vi "Test dropdown cell.vi"(11 "Test Case In":refnum<class "Test Cases.lvclass">) -> (0 "error out":errorcluster, 3 "Test Case Out":refnum<class "Test Cases.lvclass">)   [LabVIEW 2024, in "Test Cases.lvclass"]
uses:
  Test Cases.lvclass
  Test Cases.lvclass/Test Cases.ctl
  source/Grid/SourceGrid.lvclass
  <vilib>/Astemes/LUnit/Test Case.lvclass
  source/Cells/Cell/Cell.lvclass
  source/Views/Cell View/Cell View.lvclass
  source/System.Drawing.Color.ctl
  source/SourceGrid.lvlib
  source/Editors/Combo Box/Combo Box.lvclass
  C:/Program Files/National Instruments/LabVIEW 2025/vi.lib/Astemes/LUnit/Test Case.lvclass
  C:/Program Files/National Instruments/LabVIEW 2025/vi.lib/Astemes/LUnit/LUnit Runnable.lvclass
  D:/git/Sourcegrid-LabVIEW/tests/Tests/Test Cases.lvclass
  D:/git/Sourcegrid-LabVIEW/source/Editors/Editor Base/Editor Control Base.lvclass
  D:/git/Sourcegrid-LabVIEW/source/Editors/Combo Box/Combo Box.lvclass
  D:/git/Sourcegrid-LabVIEW/dll/SourceGrid.dll
  dll/SourceGrid.dll
panel:
  in  "stop":bool
  in  "Grid Container":refnum<k24>(container)
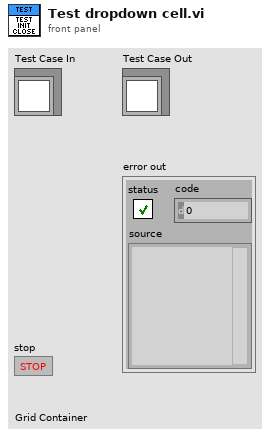
[diagram p1: front panel]
types:
  T1 = typedef "SourceGrid.lvlib/System.Drawing.Color.ctl" = enum16{"AliceBlue", "AntiqueWhite", "Aqua", "Aquamarine", "Azure", "Beige", "Bisque", "Black", "BlanchedAlmond", "Blue", "BlueViolet", "Brown", "BurlyWood", "CadetBlue", "Chartreuse", "Chocolate", "Coral", "CornflowerBlue", "Cornsilk", "Crimson", "Cyan", "DarkBlue", "DarkCyan", "DarkGoldenrod", "DarkGray", "DarkGreen", "DarkKhaki", "DarkMagenta", "DarkOliveGreen", "DarkOrange", "DarkOrchid", "DarkRed", "DarkSalmon", "DarkSeaGreen", "DarkSlateBlue", "DarkSlateGray", "DarkTurquoise", "DarkViolet", "DeepPink", "DeepSkyBlue", "DimGray", "DodgerBlue", "Firebrick", "FloralWhite", "ForestGreen", "Fuchsia", "Gainsboro", "GhostWhite", "Gold", "Goldenrod", "Gray", "Green", "GreenYellow", "Honeydew", "HotPink", "IndianRed", "Indigo", "Ivory", "Khaki", "Lavender", "LavenderBlush", "LawnGreen", "LemonChiffon", "LightBlue", "LightCoral", "LightCyan", "LightGoldenrodYellow", "LightGray", "LightGreen", "LightPink", "LightSalmon", "LightSeaGreen", "LightSkyBlue", "LightSlateGray", "LightSteelBlue", "LightYellow", "Lime", "LimeGreen", "Linen", "Magenta", "Maroon", "MediumAquamarine", "MediumBlue", "MediumOrchid", "MediumPurple", "MediumSeaGreen", "MediumSlateBlue", "MediumSpringGreen", "MediumTurquoise", "MediumVioletRed", "MidnightBlue", "MintCream", "MistyRose", "Moccasin", "NavajoWhite", "Navy", "OldLace", "Olive", "OliveDrab", "Orange", "OrangeRed", "Orchid", "PaleGoldenrod", "PaleGreen", "PaleTurquoise", "PaleVioletRed", "PapayaWhip", "PeachPuff", "Peru", "Pink", "Plum", "PowderBlue", "Purple", "Red", "RosyBrown", "RoyalBlue", "SaddleBrown", "Salmon", "SandyBrown", "SeaGreen", "SeaShell", "Sienna", "Silver", "SkyBlue", "SlateBlue", "SlateGray", "Snow", "SpringGreen", "SteelBlue", "Tan", "Teal", "Thistle", "Tomato", "Transparent", "Turquoise", "Violet", "Wheat", "White", "WhiteSmoke", "Yellow"}
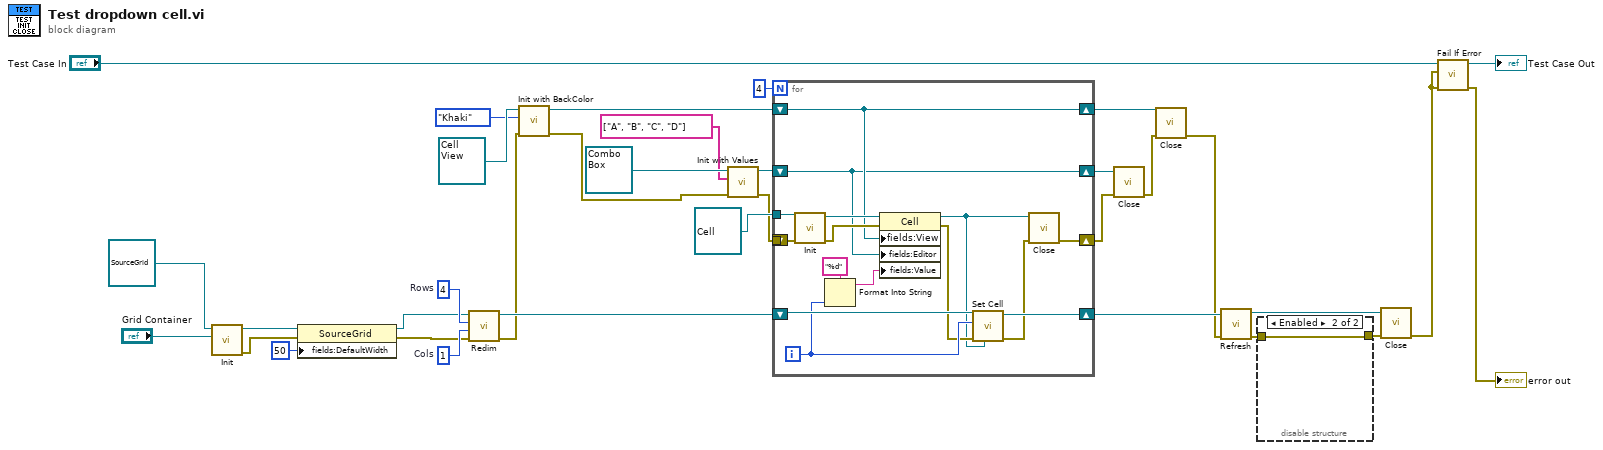
[diagram p0: block diagram]
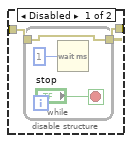
[diagram p2: hidden frame]
diagram:
  w30 = 1  # Cols
  w31 = 4  # Rows
  n1 = call-dynamic "Init.vi"("Sourcegrid Container"="Grid Container", "Grid in"=refnum<class "SourceGrid.lvclass"> refnum) -> ("error out"=w18:errorcluster, "Grid out"=w27:refnum<class "SourceGrid.lvclass">)  [unwired: 8 in]
  n2 = property class="SourceGrid"(reference=w27, error in=w18, "fields:DefaultWidth"=50 ("DefaultWidth")) -> (reference out=w26:refnum<class "SourceGrid.lvclass">, error out=w25:errorcluster)
  n3 = call "Redim.vi"("error in"=w25, "Columns"=w30, "Rows"=w31, "Sourcegrid in"=w26) -> ("error out"=w4:errorcluster, "Sourcegrid out"=w22:refnum<class "SourceGrid.lvclass">)  [unwired: 6 in]
  n4 = call-dynamic "Init with BackColor.vi"("error in"=w4, "Color"=System.Drawing.Color."Khaki", "Cell View in"=refnum<class "Cell View.lvclass"> refnum) -> ("error out"=w14:errorcluster, "Cell View out"=w6:refnum<class "Cell View.lvclass">)  [unwired: 7 in]
  n5 = call-dynamic "Init with Values.vi"("error in"=w14, "Values"=string[] ["A", "B", "C", "D"], "Combo Box in"=refnum<class "Combo Box.lvclass"> refnum ("SourceGrid.lvlib:Combo Box.lvclass")) -> ("error out"=w9:errorcluster, "Combo Box out"=w11:refnum<class "Combo Box.lvclass">)  [unwired: 7 in]
  n6 = for {
    N: 4 -> [_]
    shift-right: [w47] -> w3
    shift-left: _ -> [_]
    shift-right: [w49] -> w23
    shift-left: w22 -> [w48]
    tunnel: refnum<class "Cell.lvclass"> refnum ("Cell in") -> [w41]
    tunnel: w9 -> [w44]
    shift-right: [w37] -> w5
    shift-left: w6 -> [w37]
    shift-right: [w36] -> w1
    shift-left: w11 -> [w36]
    i -> [w45]
    n7 = call-dynamic "Init.vi"("error in"=w44, "Cell in"=w41) -> ("error out"=w39:errorcluster, "Cell out"=w40:refnum<class "Cell.lvclass">)  [unwired: 8 in]
    n8 = Format Into String(format string="%d", w45) -> (resulting string=w38:string)  [unwired: 2 in, 1 out]
    n9 = property class="Cell"(reference=w40, error in=w39, "fields:View"=w37, "fields:Editor"=w36, "fields:Value"=w38) -> (reference out=w35:refnum<class "Cell.lvclass">, error out=w42:errorcluster)
    n10 = call "Set Cell.vi"("Cell"=w35, "error in"=w42, "Row"=w45, "Sourcegrid in"=w48) -> ("error out"=w43:errorcluster, "Sourcegrid out"=w49:refnum<class "SourceGrid.lvclass">)  [unwired: 6 in]
    n11 = call-dynamic "Close.vi"("error in"=w43, "Cell in"=w35) -> ("error out"=w47:errorcluster)  [unwired: 8 in, 1 out]
  }
  n12 = call-dynamic "Close.vi"("error in"=w3, "Combo Box in"=w1) -> ("error out"=w2:errorcluster)  [unwired: 8 in, 1 out]
  n13 = call-dynamic "Close.vi"("error in"=w2, "Cell View in"=w5) -> ("error out"=w13:errorcluster)  [unwired: 8 in, 1 out]
  n14 = call "Refresh.vi"("error in"=w13, "SourceGrid in"=w23) -> ("error out"=w8:errorcluster, "SourceGrid out"=w20:refnum<class "SourceGrid.lvclass">)  [unwired: 8 in]
  n15 = disable-structure shown="Enabled" {
    disable-tunnel: w8 -> [w51 w55]
    disable-tunnel: [w50 w55] -> w7
    frame Disabled {
      n16 = while {
        tunnel: w51 -> [w52]
        tunnel: [w52] -> w50
        stop <- "stop" stop-if-true
        n17 = Wait (ms)(milliseconds to wait=u32 1) -> ()  [unwired: 1 out]
      }
    }
    frame Enabled {
    }
  }
  n18 = call-dynamic "Close.vi"("error in"=w7, "Sourcegrid in"=w20) -> ("error out"=w29:errorcluster)  [unwired: 8 in, 1 out]
  n19 = call <vilib>:"Fail If Error.vi"("error in (no error)"=w29, "Assert error"=w29, "LUnit Test Case In"="Test Case In") -> ("error out"=→"error out":errorcluster, "LUnit Test Case Out"=→"Test Case Out":refnum<class "Test Cases.lvclass">)  [unwired: 7 in]
